vi "Get Class.vi"(7 "error if not found":bool=TRUE, 8 "error in (no error)":errorcluster, 10 "class name":string, 11 "project in":refnum<vi>) -> (0 "error out":errorcluster, 1 "found":bool, 2 "class item":refnum<vi>, 3 "project out":refnum<vi>)   [LabVIEW 2021, in "MeasurementService Editor.lvlib"]
uses:
  MeasurementService Editor.lvlib
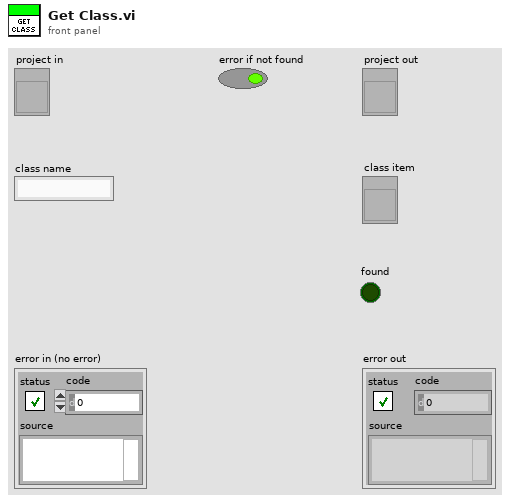
[diagram p1: front panel]
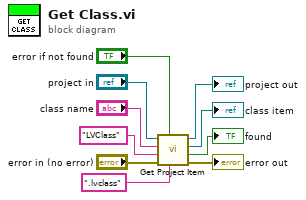
[diagram p0: block diagram]
diagram:
  n1 = call "Get Project Item.vi"("library file extension"=".lvclass", "error if not found"="error if not found", "error in (no error)"="error in (no error)", "library type"="LVClass", "library name"="class name", "project in"="project in") -> ("error out"=→"error out":errorcluster, "found"=→"found":bool, "library item"=→"class item":refnum<vi>, "project out"=→"project out":refnum<vi>)  [unwired: 2 in]
